vi "Concatenate GXML Strings.vi"() -> ()   [LabVIEW 2009]
doc: "This example demonstrates how multiple modules can share one GXML string."
uses:
  _subVIis/GXML SearchParser/gxml_SearchParser.vi
panel:
  out "Scale Info":cluster{"Offset":dbl, "Sensitivity":dbl}
  out "Log Info":cluster{"Destination":path, "File Name":string}
  out "Test Info":cluster{"Enable":bool, "Test Name":string}
  out "Concatenated GXML String":string
  in  "Scale Info":cluster{"Offset":dbl, "Sensitivity":dbl}={"Offset"=0.5, "Sensitivity"=50.1}
  in  "Log Info":cluster{"Destination":path, "File Name":string}={"Destination"=path "C:/TestData", "File Name"="Test_0530"}
  in  "Test Info":cluster{"Enable":bool, "Test Name":string}={"Enable"=TRUE, "Test Name"="Collection 1"}
  # "This example demonstrates how different components of an application can all share one GXML string.\n\n\"gxml_ConcatGXMLStrings.vi\" will combine multiple GXML strings inside one top level \nelement named <GXML_Root>.  The polymorphic XML parser \"Search Parser\" has the ability to extract \nand convert only subsets of the XML string. This enables multiple modules to share to and parse \nfrom one common XML string (or file)."
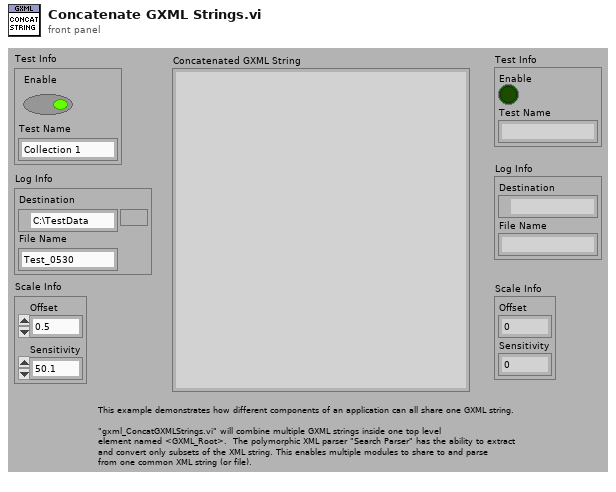
[diagram p1: front panel]
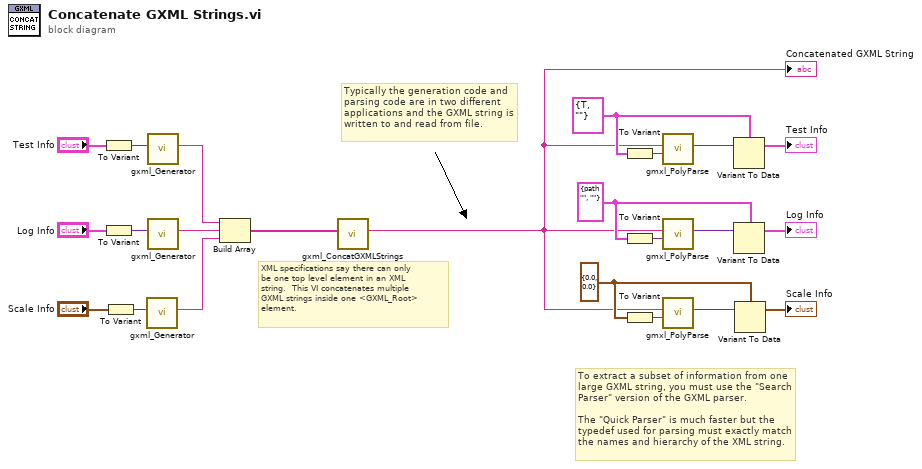
[diagram p0: block diagram]
diagram:
  w5 = cluster{"Offset":dbl, "Sensitivity":dbl} {"Offset"=0.0, "Sensitivity"=0.0} ("Scale Info")
  w6 = cluster{"Destination":path, "File Name":string} {"Destination"=path "", "File Name"=""} ("Log Info")
  w7 = cluster{"Enable":bool, "Test Name":string} {"Enable"=TRUE, "Test Name"=""} ("Test Info")
  # "Typically the generation code and parsing code are in two different applications and the GXML string is written to and read from file."
  # "XML specifications say there can only\nbe one top level element in an XML \nstring.  This VI concatenates multiple\nGXML strings inside one <GXML_Root>\nelement."
  # "To extract a subset of information from one\nlarge GXML string, you must use the \"Search \nParser\" version of the GXML parser.\n\nThe \"Quick Parser\" is much faster but the\ntypedef used for parsing must exactly match\nthe names and hierarchy of the XML string."
  n1 = To Variant(anything="Test Info") -> (Variant=w22:variant)
  n2 = To Variant(anything="Log Info") -> (Variant=w20:variant)
  n3 = To Variant(anything="Scale Info") -> (Variant=w18:variant)
  n4 = call "gxml_Generator.vi"("Variant"=w18) -> ("XML String Out"=w15:string)  [unwired: 9 in, 1 out]
  n5 = call "gxml_Generator.vi"("Variant"=w22) -> ("XML String Out"=w17:string)  [unwired: 9 in, 1 out]
  n6 = call "gxml_Generator.vi"("Variant"=w20) -> ("XML String Out"=w16:string)  [unwired: 9 in, 1 out]
  n7 = Build Array(w17, w16, w15) -> (w14:string[])
  n8 = call "gxml_ConcatGXMLStrings.vi"("GXML Strings"=w14) -> ("Concatenated GXML String"=w1:string)  [unwired: 9 in, 1 out]
  "Concatenated GXML String" <- w1
  n9 = To Variant(anything=w7) -> (Variant=w12:variant)
  n10 = To Variant(anything=w6) -> (Variant=w10:variant)
  n11 = To Variant(anything=w5) -> (Variant=w8:variant)
  n12 = call-poly "gmxl_PolyParse.vi"("TypeDesc"=w12, "XML String In"=w1) -> ("Parsed Data"=w13:variant)  [unwired: 8 in, 1 out]
  n13 = call-poly "gmxl_PolyParse.vi"("TypeDesc"=w10, "XML String In"=w1) -> ("Parsed Data"=w11:variant)  [unwired: 8 in, 1 out]
  n14 = call-poly "gmxl_PolyParse.vi"("TypeDesc"=w8, "XML String In"=w1) -> ("Parsed Data"=w9:variant)  [unwired: 8 in, 1 out]
  n15 = Variant To Data(Variant=w13, type=w7) -> (data=→"Test Info":cluster{"Enable":bool, "Test Name":string})  [unwired: 1 in, 1 out]
  n16 = Variant To Data(Variant=w11, type=w6) -> (data=→"Log Info":cluster{"Destination":path, "File Name":string})  [unwired: 1 in, 1 out]
  n17 = Variant To Data(Variant=w9, type=w5) -> (data=→"Scale Info":cluster{"Offset":dbl, "Sensitivity":dbl})  [unwired: 1 in, 1 out]
